vi "Create html index.vi"(8 "error in":errorcluster, 11 "DesignRequest":T1) -> (0 "error out":errorcluster)   [LabVIEW 2015]
uses:
  Design Request.ctl
  Variable cluster.ctl
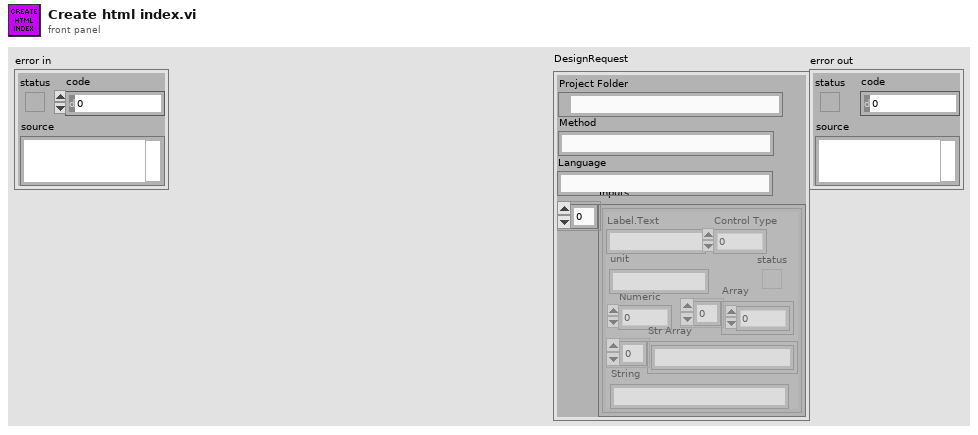
[diagram p1: front panel]
types:
  T1 = typedef "Design Request.ctl" = cluster{"Project Folder":path, "Method":string, "Inputs":T2, "Language":string}
  T2 = typedef "Variable cluster.ctl" = cluster{"Label.Text":string, "Control Type":u32, "Numeric":dbl, "Array":dbl[], "status":bool, "Str Array":string[], "String":string, "unit":string}[]
  T3 = enum16{"open", "replace", "create", "open or create", "replace or create", "replace or create with confirmation"}
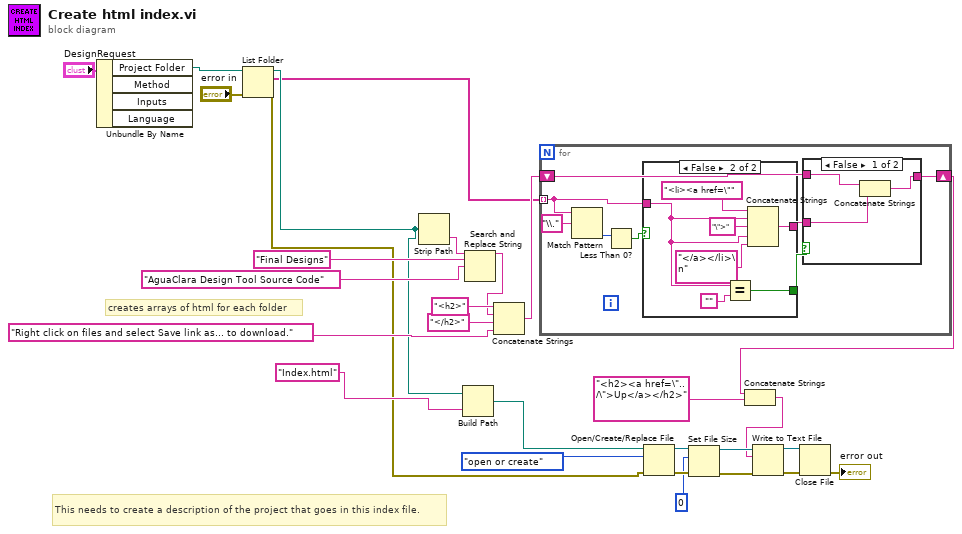
[diagram p0: block diagram]
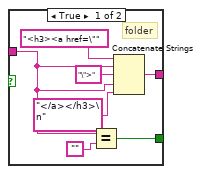
[diagram p2: hidden frame]
diagram:
  # "This needs to create a description of the project that goes in this index file."
  # "creates arrays of html for each folder"
  n1 = Unbundle By Name("DesignRequest") -> ("Project Folder"=w7:path)  [unwired: 3 out]
  n2 = List Folder(path=w7, error in="error in") -> (path out=w6:path, filenames=w5:string[], error out=w3:errorcluster)  [unwired: 2 in, 1 out]
  n3 = Strip Path(path=w6) -> (name=w11:string)  [unwired: 1 out]
  n4 = Build Path(base path=w6, name or relative path="Index.html") -> (appended path=w23:path)
  n5 = Search and Replace String(input string=w11, search string="Final Designs" ("string"), replace string="AguaClara Design Tool Source Code" ("string")) -> (result string=w10:string)  [unwired: 5 in, 3 out]
  n6 = Concatenate Strings("<h2>" ("string"), w10, "</h2>" ("string"), "Right click on files and select Save link as... to download." ("string")) -> (w12:string)
  n7 = for {
    tunnel: w5 -> [w32] mode=indexing
    shift-right: [w36] -> w9
    shift-left: w12 -> [w34]
    n8 = Match Pattern(string=w32, regular expression="\\.") -> (offset past match=w31:i32)  [unwired: 1 in, 3 out]
    n9 = Less Than 0?(x=w31) -> (x < 0?=w30:bool)
    n10 = case shown="False" w30 {
      tunnel: [w41 w48] -> w35
      tunnel: w32 -> [w38 w45]
      tunnel: [w37 w44] -> w33
      frame True {
        # "folder"
        n11 = Equal?(x=w38, y="") -> (x = y?=w37:bool)
        n12 = Concatenate Strings("<h3><a href=\"" ("string"), w38, "\">" ("string"), w38, "</a></h3>\n" ("string")) -> (w41:string)
      }
      frame False {
        n13 = Equal?(x=w45, y="") -> (x = y?=w44:bool)
        n14 = Concatenate Strings("<li><a href=\"" ("string"), w45, "\">" ("string"), w45, "</a></li>\n" ("string")) -> (w48:string)
      }
    }
    n15 = case shown="False" w33 {
      tunnel: [w53 w54] -> w36
      tunnel: w35 -> [w52 _]
      tunnel: w34 -> [w51 w54]
      frame False {
        n16 = Concatenate Strings(w51, w52) -> (w53:string)
      }
      frame True {
      }
    }
  }
  n17 = Open/Create/Replace File(file path (use dialog)=w23, error in=w3, operation (0:open)=T3."open or create") -> (refnum out=w19:refnum<file>, error out=w17:errorcluster)  [unwired: 3 in, 1 out]
  n18 = Set File Size(4:w17, 6:i64 0 ("size (in bytes)"), 7:w19) -> (0:w16:errorcluster, 3:w18:refnum<file>)
  n19 = Concatenate Strings(w9, "<h2><a href=\"../\">Up</a></h2>" ("name or relative path")) -> (w8:string)
  n20 = Write to Text File(file (use dialog)=w18, text=w8, error in=w16) -> (refnum out=w20:refnum<file>, error out=w21:errorcluster)  [unwired: 1 in, 1 out]
  n21 = Close File(refnum=w20, error in=w21) -> (error out=→"error out":errorcluster)  [unwired: 1 out]
